vi "MathUtil_InputModulus.vi"(9 "Maximum_Input":dbl, 10 "Minimum_Input":dbl, 11 "Input":dbl) -> (3 "modulus":dbl)   [LabVIEW 2019, in "Trajectory_Library.lvlib"]
doc: "Returns modulus of input. This is used for continuous systems, for example rotational systems.\n \nInputs:\n - input -- Input value to wrap.\n - minimumInput -- The minimum value expected from the input.\n - maximumInput -- The maximum value expected from the input.\n\nOutputs:\n - modulus -- The wrapped value.\n - AltModulus -- The wrapped value calculated a different way (used only for debugging).\n - Different -- If TRUE, then the modulus and AltModulus are different... (used only for debugging)"
uses:
  Trajectory_Library.lvlib
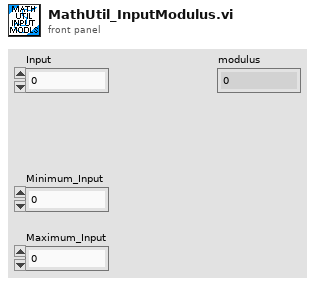
[diagram p1: front panel]
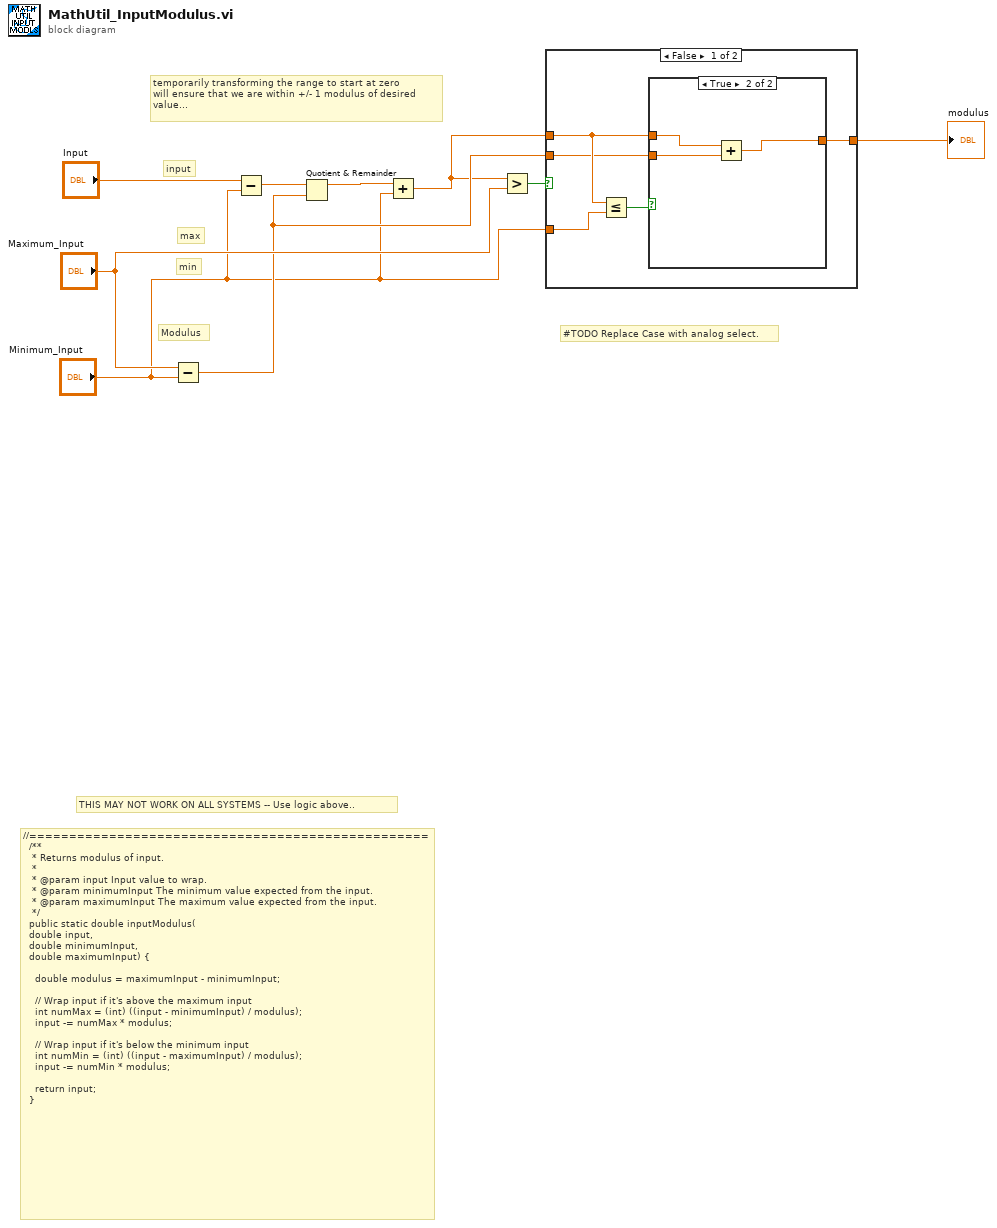
[diagram p0: block diagram]
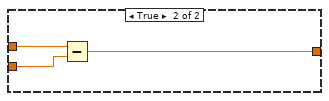
[diagram p3: hidden frame]
diagram:
  # "temporarily transforming the range to start at zero\nwill ensure that we are within +/- 1 modulus of desired\nvalue..."
  # "min"
  # "max"
  # "input"
  # "#TODO Replace Case with analog select."
  # "Modulus"
  # "THIS MAY NOT WORK ON ALL SYSTEMS -- Use logic above.."
  # "//==================================================\n  /**\n   * Returns modulus of input.\n   *\n   * @param input Input value to wrap.\n   * @param minimumInput The minimum value expected from the input.\n   * @param maximumInput The maximum value expected from the input.\n   */\n  public static double inputModulus(\n\t\tdouble input, \n\t\tdouble minimumInput, \n\t\tdouble maximumInput) {\n\n    double modulus = maximumInput - minimumInput;\n\n    // Wrap input if it's above the maximum input\n    int numMax = (int) ((input - minimumInput) / modulus);\n    input -= numMax * modulus;\n\n    // Wrap input if it's below the minimum input\n    int numMin = (int) ((input - maximumInput) / modulus);\n    input -= numMin * modulus;\n\n    return input;\n  }"
  n1 = Subtract(x="Maximum_Input", y="Minimum_Input") -> (x-y=w7:dbl)
  n2 = Subtract(x="Input", y="Minimum_Input") -> (x-y=w3:dbl)
  n3 = Quotient & Remainder(x=w3, y=w7) -> (x-y*floor(x/y)=w5:dbl)  [unwired: 1 out]
  n4 = Add(x=w5, y="Minimum_Input") -> (x+y=w4:dbl)
  n5 = Greater?(x=w4, y="Maximum_Input") -> (0:w8:bool)
  n6 = case shown="False" w8 {
    tunnel: w4 -> [w12 w21]
    tunnel: w7 -> [w11 w20]
    tunnel: [w10 w19] -> w6
    tunnel: "Minimum_Input" -> [w13 _]
    frame False {
      n7 = Less Or Equal?(x=w12, y=w13) -> (x <= y?=w14:bool)
      n8 = case shown="True" w14 {
        tunnel: w12 -> [w15 w18]
        tunnel: w11 -> [_ w17]
        tunnel: [w15 w16] -> w10
        frame False {
        }
        frame True {
          n9 = Add(x=w18, y=w17) -> (x+y=w16:dbl)
        }
      }
    }
    frame True {
      n10 = Subtract(x=w21, y=w20) -> (x-y=w19:dbl)
    }
  }
  "modulus" <- w6
